vi "Get API Interface Info.vi"(8 "error in (no error)":errorcluster, 10 "CASE":string, 11 "CSM-Helper in":refnum<class "CSM-Helper.lvclass">) -> (0 "error out":errorcluster, 1 "Response":T1, 2 "Argument":T1, 3 "CSM-Helper out":refnum<class "CSM-Helper.lvclass">)   [LabVIEW 2020, in "CSM-Helper.lvclass"]
uses:
  CSM-Helper.lvclass
  Typedef/Def-Argument Info.ctl
  CSM-Helper.lvclass/CSM-Helper.ctl
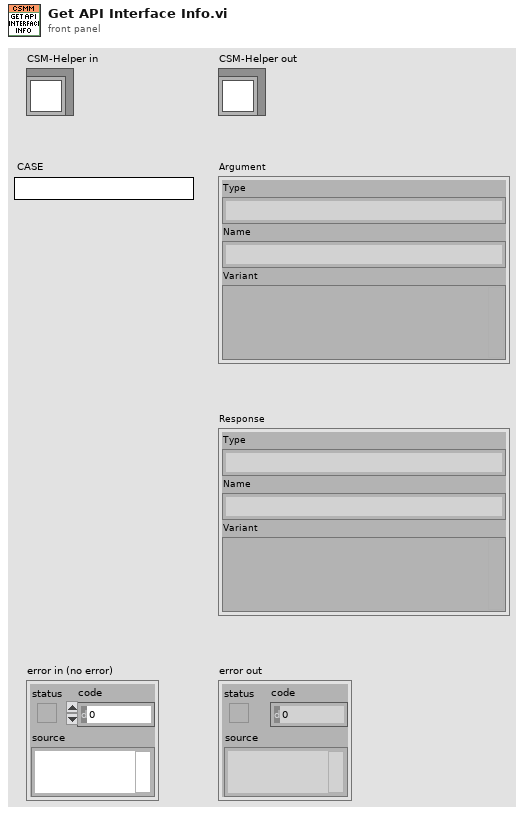
[diagram p1: front panel]
types:
  T1 = typedef "CSM-Helper.lvclass/Def-Argument Info.ctl" = cluster{"Type":string, "Name":string, "Variant":variant}
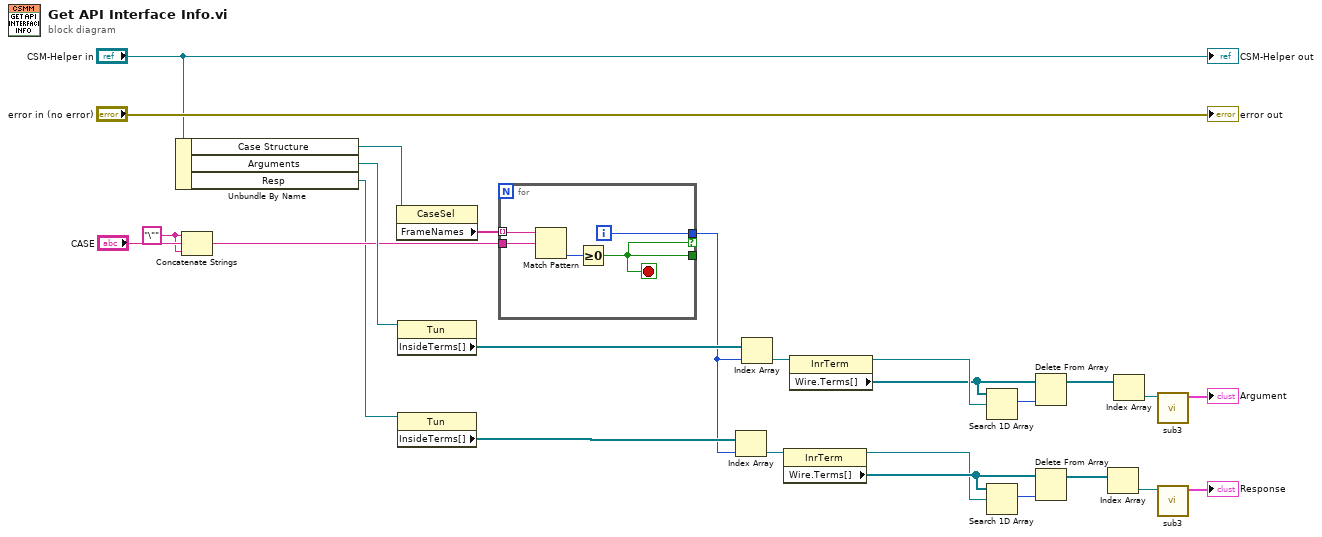
[diagram p0: block diagram]
diagram:
  w19 = "\"" ("string")
  n1 = Unbundle By Name("CSM-Helper in") -> ("Case Structure"=w24:refnum<vi>, "Arguments"=w23:refnum<vi>, "Resp"=w14:refnum<vi>)
  n2 = Concatenate Strings(w19, "CASE", w19) -> (w20:string)
  n3 = property class="CaseSel"(reference=w24) -> ("FrameNames"=w22:string[])  [unwired: 1 in, 2 out]
  n4 = property class="Tun"(reference=w23) -> ("InsideTerms[]"=w18:refnum<vi>[])  [unwired: 1 in, 2 out]
  n5 = property class="Tun"(reference=w14) -> ("InsideTerms[]"=w15:refnum<vi>[])  [unwired: 1 in, 2 out]
  n6 = for {
    tunnel: w22 -> [w31] mode=indexing
    tunnel: w20 -> [w30]
    tunnel: [w29] -> w13 if=w27
    tunnel: [w27] -> _
    i -> [w29]
    stop <- w27 stop-if-true
    n7 = Match Pattern(string=w31, regular expression=w30) -> (offset past match=w28:i32)  [unwired: 1 in, 3 out]
    n8 = Greater Or Equal To 0?(x=w28) -> (x >= 0?=w27:bool)
  }
  n9 = Index Array(array=w15, index=w13) -> (element=w11:refnum<vi>)
  n10 = Index Array(array=w18, index=w13) -> (element=w17:refnum<vi>)
  n11 = property class="InrTerm"(reference=w11) -> (reference out=w1:refnum<vi>, "Wire.Terms[]"=w2:refnum<vi>[])  [unwired: 1 in, 1 out]
  n12 = property class="InrTerm"(reference=w17) -> (reference out=w8:refnum<vi>, "Wire.Terms[]"=w7:refnum<vi>[])  [unwired: 1 in, 1 out]
  n13 = Search 1D Array(1D array=w7, element=w8) -> (index of element=w6:i32)  [unwired: 1 in]
  n14 = Search 1D Array(1D array=w2, element=w1) -> (index of element=w4:i32)  [unwired: 1 in]
  n15 = Delete From Array(array=w7, index=w6) -> (array with subset deleted=w5:refnum<vi>[])  [unwired: 1 in, 1 out]
  n16 = Delete From Array(array=w2, index=w4) -> (array with subset deleted=w3:refnum<vi>[])  [unwired: 1 in, 1 out]
  n17 = Index Array(array=w3) -> (element=w9:refnum<vi>)  [unwired: 1 in]
  n18 = Index Array(array=w5) -> (element=w16:refnum<vi>)  [unwired: 1 in]
  n19 = call "sub3.vi"("Terminal in"=w16) -> ("Argument"=→"Argument":T1)  [unwired: 10 in]
  n20 = call "sub3.vi"("Terminal in"=w9) -> ("Argument"=→"Response":T1)  [unwired: 10 in]
  "error out" <- "error in (no error)"
  "CSM-Helper out" <- "CSM-Helper in"
